vi "Planta_303_ver2.vi"() -> ()   [LabVIEW 2014]
uses:
  <vilib>/measure/NI_MABase.lvlib
panel:
  out "Tank 2":dbl(slide) scale=0.0..10.0
  out "Tank":dbl(slide) scale=0.0..200.0
  in  "Escolha o Sinal":string(combo)
  out "Waveform Chart":waveform(dbl)(graph)
  in  "Amplitude":dbl=1.0
  in  "Frequency":dbl=10.1
  in  "Offset":dbl
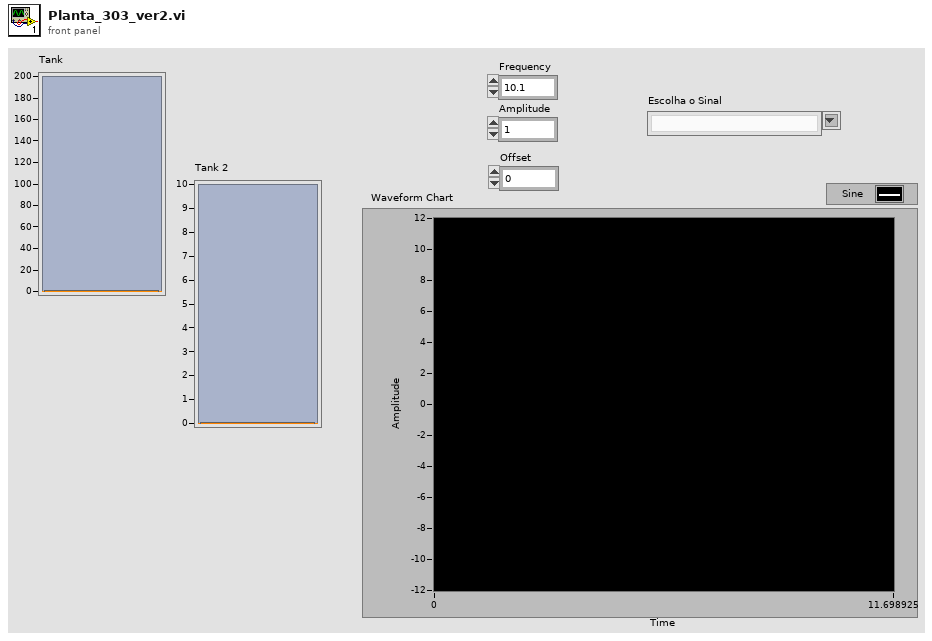
[diagram p1: front panel]
types:
  T1 = enum16{"Sine Wave", "Triangle Wave", "Square Wave", "Sawtooth Wave"}
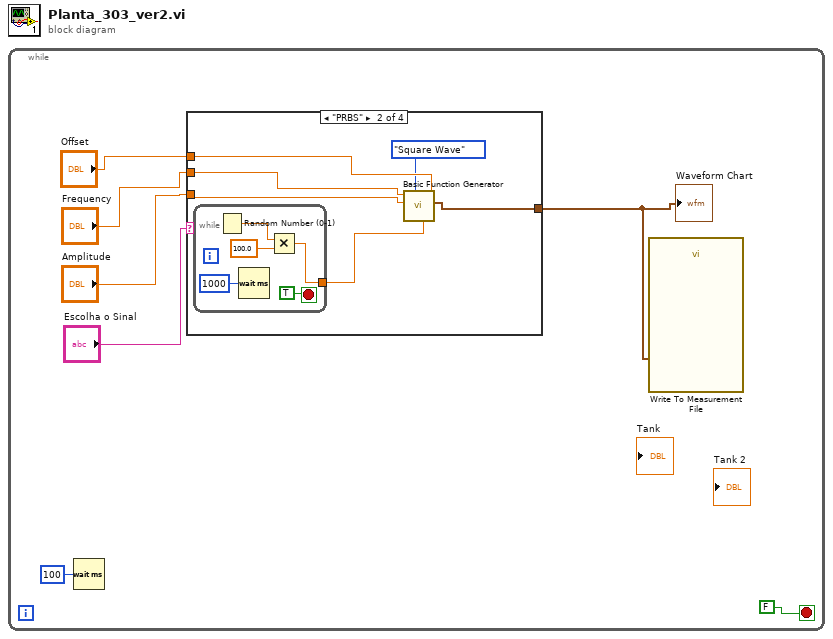
[diagram p0: block diagram]
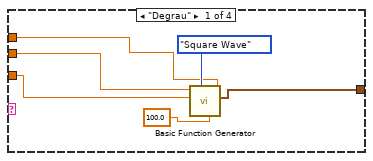
[diagram p2: hidden frame]
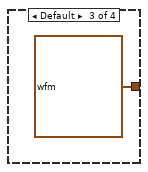
[diagram p3: hidden frame]
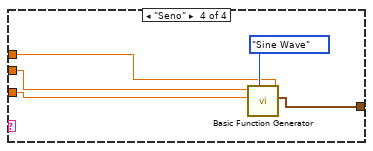
[diagram p4: hidden frame]
diagram:
  n1 = while {
    stop <- FALSE stop-if-true
    n2 = Wait (ms)(milliseconds to wait=u32 100) -> ()  [unwired: 1 out]
    n3 = case shown="\"PRBS\"" "Escolha o Sinal" {
      tunnel: "Offset" -> [w12 w17 _ w29]
      tunnel: "Frequency" -> [w10 w16 _ w28]
      tunnel: "Amplitude" -> [w9 w18 _ w27]
      tunnel: [w8 w19 waveform(dbl) {"t0"=timestamp(0 s since 1904-01-01), "dt"=1.0, "Y"=[]} ("signal out") w26] -> w2
      frame "Degrau" {
        n4 = call <vilib>:"Basic Function Generator.vi"("offset"=w12, "square wave duty cycle (%)"=100.0 ("Duty Cycle (%)"), "signal type"=T1."Square Wave", "amplitude"=w9, "frequency"=w10) -> ("signal out"=w8:waveform(dbl))  [unwired: 4 in, 2 out]
      }
      frame "PRBS" {
        n5 = while {
          tunnel: [w23] -> w15
          stop <- TRUE stop-if-true
          n6 = Random Number (0-1)() -> (number: 0 to 1=w24:dbl)
          n7 = Wait (ms)(milliseconds to wait=u32 1000) -> ()  [unwired: 1 out]
          n8 = Multiply(x=w24, y=100.0) -> (x*y=w23:dbl)
        }
        n9 = call <vilib>:"Basic Function Generator.vi"("offset"=w17, "square wave duty cycle (%)"=w15, "signal type"=T1."Square Wave", "amplitude"=w18, "frequency"=w16) -> ("signal out"=w19:waveform(dbl))  [unwired: 4 in, 2 out]
      }
      frame Default {
      }
      frame "Seno" {
        n10 = call <vilib>:"Basic Function Generator.vi"("offset"=w29, "signal type"=T1."Sine Wave", "amplitude"=w27, "frequency"=w28) -> ("signal out"=w26:waveform(dbl))  [unwired: 5 in, 2 out]
      }
    }
    "Waveform Chart" <- w2
    n11 = call "Write To Measurement File"("Signals"=w2) -> ()  [unwired: 16 in, 3 out]
  }
